vi "Build String days.vi"(11 "Weekday filter":T1) -> (3 "output string":string)   [LabVIEW 2018]
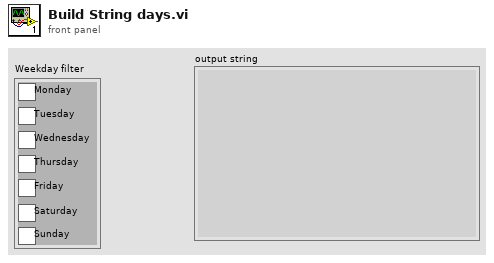
[diagram p1: front panel]
types:
  T1 = cluster{"Monday":bool, "Tuesday":bool, "Wednesday":bool, "Thursday":bool, "Friday":bool, "Saturday":bool, "Sunday":bool}
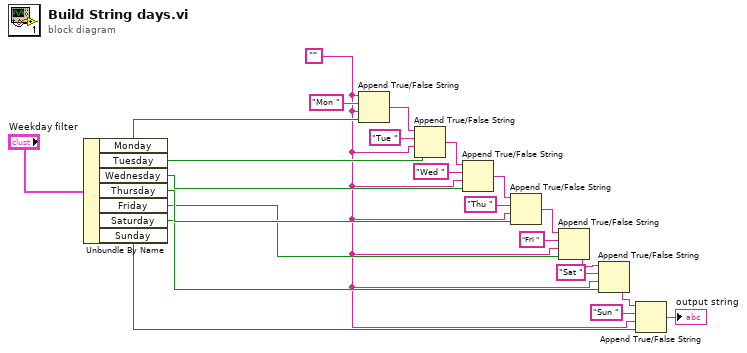
[diagram p0: block diagram]
diagram:
  w2 = ""
  n1 = Unbundle By Name("Weekday filter") -> ("Monday"=w22:bool, "Tuesday"=w8:bool, "Wednesday"=w7:bool, "Thursday"=w6:bool, "Friday"=w5:bool, "Saturday"=w4:bool, "Sunday"=w3:bool)
  n2 = Append True/False String(1:w22, 2:w2, 3:"Mon " ("true string"), 4:w2) -> (0:w15:string)
  n3 = Append True/False String(1:w8, 2:w2, 3:"Tue " ("true string"), 4:w15) -> (0:w14:string)
  n4 = Append True/False String(1:w7, 2:w2, 3:"Wed " ("true string"), 4:w14) -> (0:w13:string)
  n5 = Append True/False String(1:w6, 2:w2, 3:"Thu " ("true string"), 4:w13) -> (0:w12:string)
  n6 = Append True/False String(1:w5, 2:w2, 3:"Fri " ("true string"), 4:w12) -> (0:w11:string)
  n7 = Append True/False String(1:w4, 2:w2, 3:"Sat " ("true string"), 4:w11) -> (0:w9:string)
  n8 = Append True/False String(1:w3, 2:w2, 3:"Sun " ("true string"), 4:w9) -> (0:→"output string":string)
